vi "AIT 664 - Parse Tree Parameters.vi"(0 "Item Ref in":T1 format="%.0x", 2 "Access Type":T2=enum."Write", 11 "error in":errorcluster) -> (6 "Parameter References out":T1[](array[typedef]) format="%.0x", 8 "Queue Transmit Channel out":T1=18446744073709551615 format="%.0x", 10 "Parameter Driver Data out":T3 {"Num Bits" min=1 max=32}, 15 "error out":errorcluster)   [LabVIEW 2013, in "AIT 664 Custom Device.lvlib"]
doc: "Given the user defined channels from Veristand (first byte, start bit, number of bits, etc) gather that information to be able to convert between the U8 array of data from the AIT 664 card and the Veristand double array.\n\nAdditionally, grab Veristand references to each of the channels and status information, (timestamp, network, etc for reads, transmit for writes) so we can obtain a block data reference from Veristand. When we decide to move data from the driver to veristand we'll supply the double array of channels and status and the block data reference and Veristand will mate the two and present them to the user."
uses:
  AIT 664 Custom Device.lvlib
  <vilib>/NI Veristand/Custom Device API/Custom Device Item Ref.ctl
  RT Controls/AIT 664 - Driver Data.ctl
  Controls and Global/Start Bit.ctl
  Controls and Global/Number of Bits.ctl
  <vilib>/NI Veristand/Custom Device API/Data Access Type.ctl
  <vilib>/NI Veristand/Custom Device Tools/Custom Device Utility Library/NI VeriStand - Search for All Items by GUID.vi
  Controls and Global/Global.vi
  <vilib>/NI Veristand/Custom Device API/Get Item Property (Double).vi
  <vilib>/NI Veristand/Custom Device API/Get Item Property (Boolean).vi
  <vilib>/NI Veristand/Custom Device API/Get Item Property (I32).vi
  <vilib>/NI Veristand/Custom Device Tools/Custom Device Utility Library/NI VeriStand - Search for Item by GUID.vi
  <vilib>/NI Veristand/Custom Device API/Custom Device API.lvlib
  <vilib>/NI Veristand/Custom Device Tools/Custom Device Utility Library/Custom Device Utility Library.lvlib
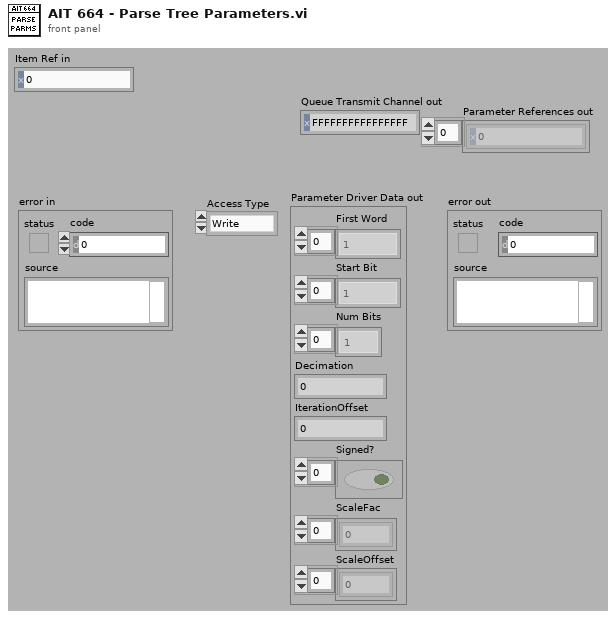
[diagram p1: front panel]
types:
  T1 = typedef "Custom Device API.lvlib/Custom Device Item Ref.ctl" = u64
  T2 = typedef "Custom Device API.lvlib/Data Access Type.ctl" = enum16{"Read", "Write"}
  T3 = typedef "AIT 664 Custom Device.lvlib/AIT 664 - Driver Data.ctl" = cluster{"First Word":T4[], "Start Bit":T4[], "Num Bits":T5[], "Decimation":i32, "IterationOffset":i32, "Signed?":bool[], "ScaleFac":dbl[], "ScaleOffset":dbl[]}
  T4 = typedef "AIT 664 Custom Device.lvlib/Start Bit.ctl" = i32
  T5 = typedef "AIT 664 Custom Device.lvlib/Number of Bits.ctl" = i32
  T6 = typedef "Custom Device API.lvlib/Custom Device Item Info.ctl" = cluster{"Name":string, "Is Channel":bool, "GUID":string, "Is Waveform":bool}
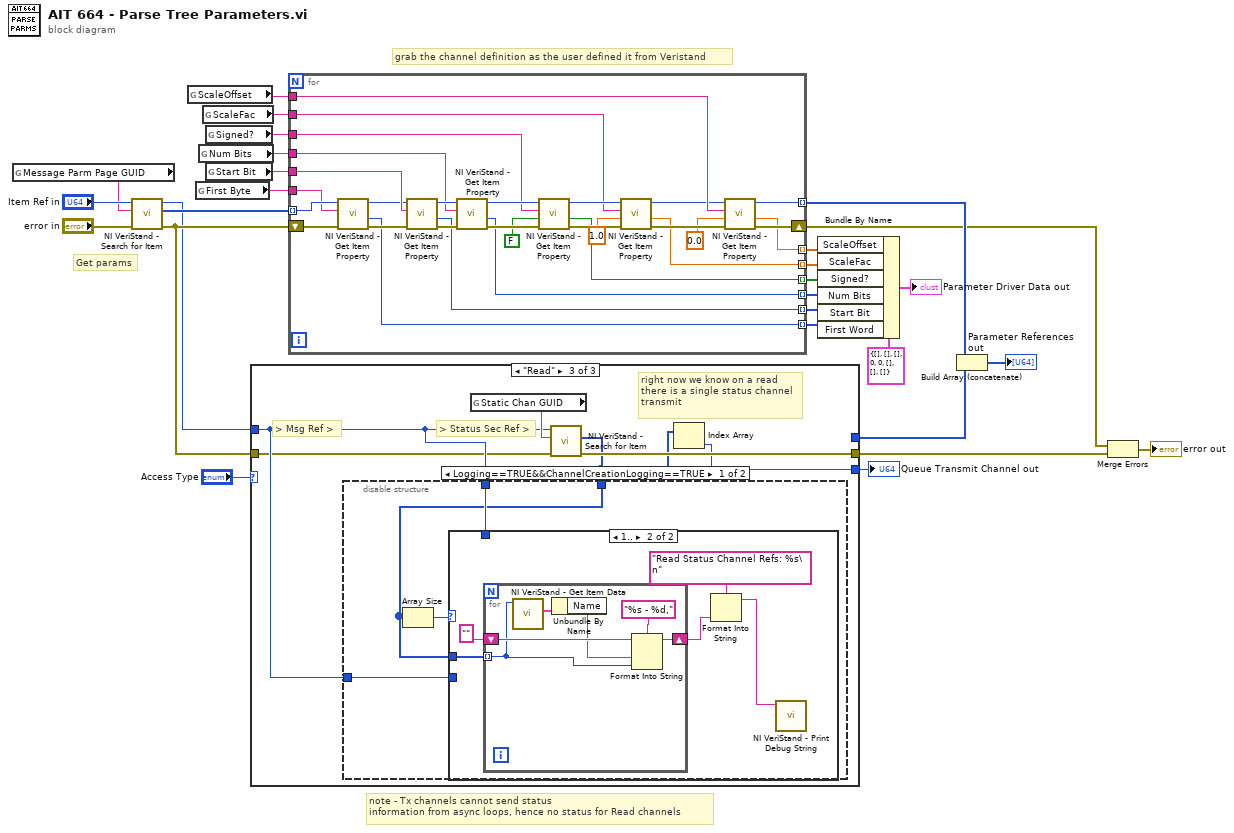
[diagram p0: block diagram]
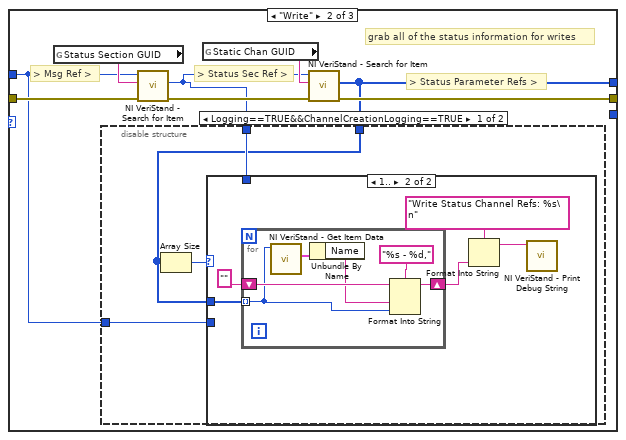
[diagram p3: hidden frame]
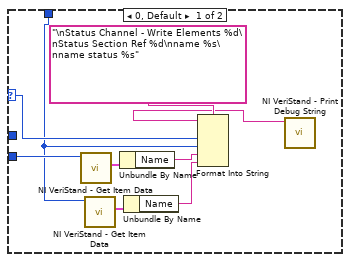
[diagram p4: hidden frame]
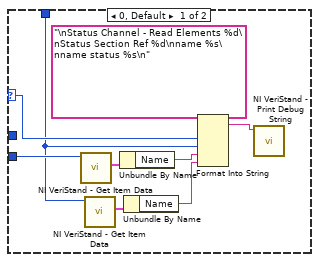
[diagram p6: hidden frame]
diagram:
  # "grab the channel definition as the user defined it from Veristand"
  # "note - Tx channels cannot send status\ninformation from async loops, hence no status for Read channels"
  # "Get params"
  n1 = global read "Global.vi" "Message Parm Page GUID"() -> (w8:string)
  n2 = call-poly <vilib>:"NI VeriStand - Search for Item.vi"("error in"="error in", "Item GUID"=w8, "Section Ref in"="Item Ref in") -> ("error out"=w12:errorcluster, "Item Refs"=w7:T1[], "Section Ref out"=w5:T1)  [unwired: 5 in, 1 out]
  n3 = global read "Global.vi" "ScaleOffset"() -> (w22:string)
  n4 = global read "Global.vi" "First Byte"() -> (w19:string)
  n5 = global read "Global.vi" "Num Bits"() -> (w28:string)
  n6 = global read "Global.vi" "ScaleFac"() -> (w23:string)
  n7 = global read "Global.vi" "Signed?"() -> (w24:string)
  n8 = global read "Global.vi" "Start Bit"() -> (w27:string)
  n9 = case shown="\"Read\"" "Access Type" {
    tunnel: w5 -> [_ w30 w65]
    tunnel: w12 -> [w29 w37 w64]
    tunnel: [w29 w33 w66] -> w11
    tunnel: [_ w31 _] -> w9
    tunnel: [_ _ w62] -> w1
    frame Default {
    }
    frame "Write" {
      # "grab all of the status information for writes"
      # "> Status Parameter Refs >"
      # "> Status Sec Ref >"
      # "> Msg Ref >"
      n10 = global read "Global.vi" "Status Section GUID"() -> (w36:string)
      n11 = call-poly <vilib>:"NI VeriStand - Search for Item.vi"("error in"=w37, "Item GUID"=w36, "Section Ref in"=w30) -> ("error out"=w35:errorcluster, "Item Ref"=w32:T1)  [unwired: 5 in, 2 out]
      n12 = global read "Global.vi" "Static Chan GUID"() -> (w34:string)
      n13 = call-poly <vilib>:"NI VeriStand - Search for Item.vi"("error in"=w35, "Item GUID"=w34, "Section Ref in"=w32) -> ("error out"=w33:errorcluster, "Item Refs"=w31:T1[])  [unwired: 5 in, 2 out]
      n14 = disable-structure shown="Logging==TRUE&&ChannelCreationLogging==TRUE" {
        disable-tunnel: w31 -> [w39 _]
        disable-tunnel: w32 -> [w40 _]
        disable-tunnel: w30 -> [w38 _]
        frame condition #0 (active) {
          n15 = Array Size(array=w39) -> (size(s)=w41:i32)
          n16 = case shown="1.." w41 {
            selector: w41 -> [w49 _]
            tunnel: w39 -> [_ w54]
            tunnel: w40 -> [w45 _]
            tunnel: w38 -> [w47 _]
            frame 0, Default {
              n17 = call <vilib>:"NI VeriStand - Get Item Data.vi"("Item Ref in"=w47) -> ("Item Info"=w48:T6)  [unwired: 7 in, 3 out]
              n18 = call <vilib>:"NI VeriStand - Get Item Data.vi"("Item Ref in"=w45) -> ("Item Info"=w46:T6)  [unwired: 7 in, 3 out]
              n19 = Unbundle By Name(w48) -> ("Name"=w44:string)
              n20 = Unbundle By Name(w46) -> ("Name"=w43:string)
              n21 = Format Into String(format string="\nStatus Channel - Write Elements %d\nStatus Section Ref %d\nname %s\nname status %s" ("Debug String"), w49, w45, w44, w43) -> (resulting string=w42:string)  [unwired: 2 in, 1 out]
              n22 = call <vilib>:"NI VeriStand - Print Debug String.vi"("Message"=w42) -> ()  [unwired: 10 in, 1 out]
            }
            frame 1.. {
              n23 = for {
                tunnel: w54 -> [w58] mode=indexing
                shift-right: [w59] -> w52
                shift-left: "" ("format string") -> [w60]
                n24 = call <vilib>:"NI VeriStand - Get Item Data.vi"("Item Ref in"=w58) -> ("Item Info"=w57:T6)  [unwired: 7 in, 3 out]
                n25 = Unbundle By Name(w57) -> ("Name"=w56:string)
                n26 = Format Into String(format string="%s - %d,", initial string=w60, w56, w58) -> (resulting string=w59:string)  [unwired: 1 in, 1 out]
              }
              n27 = Format Into String(format string="Write Status Channel Refs: %s\n", w52) -> (resulting string=w51:string)  [unwired: 2 in, 1 out]
              n28 = call <vilib>:"NI VeriStand - Print Debug String.vi"("Message"=w51) -> ()  [unwired: 10 in, 1 out]
            }
          }
        }
        frame condition #1 {
        }
      }
    }
    frame "Read" {
      # "right now we know on a read\nthere is a single status channel\ntransmit"
      # "> Status Sec Ref >"
      # "> Msg Ref >"
      n29 = global read "Global.vi" "Static Chan GUID"() -> (w67:string)
      n30 = call-poly <vilib>:"NI VeriStand - Search for Item.vi"("error in"=w64, "Item GUID"=w67, "Section Ref in"=w65) -> ("error out"=w66:errorcluster, "Item Refs"=w63:T1[])  [unwired: 5 in, 2 out]
      n31 = disable-structure shown="Logging==TRUE&&ChannelCreationLogging==TRUE" {
        disable-tunnel: w63 -> [w69 _]
        disable-tunnel: w65 -> [w70 _]
        disable-tunnel: w65 -> [w68 _]
        frame condition #0 (active) {
          n32 = Array Size(array=w69) -> (size(s)=w71:i32)
          n33 = case shown="1.." w71 {
            selector: w71 -> [w79 _]
            tunnel: w69 -> [_ w84]
            tunnel: w70 -> [w75 _]
            tunnel: w68 -> [w77 _]
            frame 0, Default {
              n34 = call <vilib>:"NI VeriStand - Get Item Data.vi"("Item Ref in"=w77) -> ("Item Info"=w78:T6)  [unwired: 7 in, 3 out]
              n35 = call <vilib>:"NI VeriStand - Get Item Data.vi"("Item Ref in"=w75) -> ("Item Info"=w76:T6)  [unwired: 7 in, 3 out]
              n36 = Unbundle By Name(w78) -> ("Name"=w74:string)
              n37 = Unbundle By Name(w76) -> ("Name"=w73:string)
              n38 = Format Into String(format string="\nStatus Channel - Read Elements %d\nStatus Section Ref %d\nname %s\nname status %s\n" ("Debug String"), w79, w75, w74, w73) -> (resulting string=w72:string)  [unwired: 2 in, 1 out]
              n39 = call <vilib>:"NI VeriStand - Print Debug String.vi"("Message"=w72) -> ()  [unwired: 10 in, 1 out]
            }
            frame 1.. {
              n40 = for {
                tunnel: w84 -> [w88] mode=indexing
                shift-right: [w89] -> w82
                shift-left: "" ("format string") -> [w90]
                n41 = call <vilib>:"NI VeriStand - Get Item Data.vi"("Item Ref in"=w88) -> ("Item Info"=w87:T6)  [unwired: 7 in, 3 out]
                n42 = Unbundle By Name(w87) -> ("Name"=w86:string)
                n43 = Format Into String(format string="%s - %d,", initial string=w90, w86, w88) -> (resulting string=w89:string)  [unwired: 1 in, 1 out]
              }
              n44 = Format Into String(format string="Read Status Channel Refs: %s\n", w82) -> (resulting string=w81:string)  [unwired: 2 in, 1 out]
              n45 = call <vilib>:"NI VeriStand - Print Debug String.vi"("Message"=w81) -> ()  [unwired: 10 in, 1 out]
            }
          }
        }
        frame condition #1 {
        }
      }
      n46 = Index Array(array=w63) -> (element=w62:T1)  [unwired: 1 in]
    }
  }
  "Queue Transmit Channel out" <- w1
  n47 = for {
    shift-right: [w112] -> w2
    shift-left: w12 -> [w105]
    tunnel: w7 -> [w104] mode=indexing
    tunnel: w27 -> [w118]
    tunnel: w28 -> [w117]
    tunnel: [w116] -> w17 mode=indexing
    tunnel: [w113] -> w4 mode=indexing
    tunnel: w24 -> [w108]
    tunnel: w23 -> [w99]
    tunnel: w22 -> [w100]
    tunnel: w19 -> [w103]
    tunnel: [w98] -> w18 mode=indexing
    tunnel: [w97] -> w16 mode=indexing
    tunnel: [w96] -> w15 mode=indexing
    tunnel: [w94] -> w14 mode=indexing
    tunnel: [w93] -> w13 mode=indexing
    n48 = call-poly <vilib>:"NI VeriStand - Get Item Property.vi"("error in (no error)"=w105, "Property Name"=w103, "Item Ref in"=w104) -> ("error out"=w101:errorcluster, "Value"=w98:i32, "Item Ref out"=w102:T1)  [unwired: 5 in, 1 out]
    n49 = call-poly <vilib>:"NI VeriStand - Get Item Property.vi"("error in (no error)"=w101, "Property Name"=w118, "Item Ref in"=w102) -> ("error out"=w120:errorcluster, "Value"=w116:i32, "Item Ref out"=w119:T1)  [unwired: 5 in, 1 out]
    n50 = call-poly <vilib>:"NI VeriStand - Get Item Property.vi"("error in (no error)"=w120, "Property Name"=w117, "Item Ref in"=w119) -> ("error out"=w109:errorcluster, "Value"=w97:i32, "Item Ref out"=w115:T1)  [unwired: 5 in, 1 out]
    n51 = call-poly <vilib>:"NI VeriStand - Get Item Property.vi"("error in (no error)"=w109, "Default Value"=FALSE, "Property Name"=w108, "Item Ref in"=w115) -> ("error out"=w110:errorcluster, "Value"=w96:bool, "Item Ref out"=w114:T1)  [unwired: 4 in, 1 out]
    n52 = call-poly <vilib>:"NI VeriStand - Get Item Property.vi"("error in (no error)"=w110, "Default Value"=1.0, "Property Name"=w99, "Item Ref in"=w114) -> ("error out"=w111:errorcluster, "Value"=w94:dbl, "Item Ref out"=w92:T1)  [unwired: 4 in, 1 out]
    n53 = call-poly <vilib>:"NI VeriStand - Get Item Property.vi"("error in (no error)"=w111, "Default Value"=0.0, "Property Name"=w100, "Item Ref in"=w92) -> ("error out"=w112:errorcluster, "Value"=w93:dbl, "Item Ref out"=w113:T1)  [unwired: 4 in, 1 out]
  }
  n54 = Bundle By Name(cluster=T3 {"First Word"=[], "Start Bit"=[], "Num Bits"=[], "Decimation"=0, "IterationOffset"=0, "Signed?"=[], "ScaleFac"=[], "ScaleOffset"=[]} ("Parameter Driver Data"), "ScaleOffset"=w13, "ScaleFac"=w14, "Signed?"=w15, "Num Bits"=w16, "Start Bit"=w17, "First Word"=w18) -> (→"Parameter Driver Data out":T3)
  n55 = Build Array (concatenate)(w4, w9) -> (→"Parameter References out":T1[])
  n56 = Merge Errors(w2, w11) -> (→"error out":errorcluster)
